vi "ChangePBTime.vi"(8 "Instruction to change":i32, 9 "Time":dbl, 10 "Input parameters":T2) -> (1 "Time out":dbl, 2 "output parameters":T2)   [LabVIEW 2013]
uses:
  6704/6704_static_voltages_control.ctl
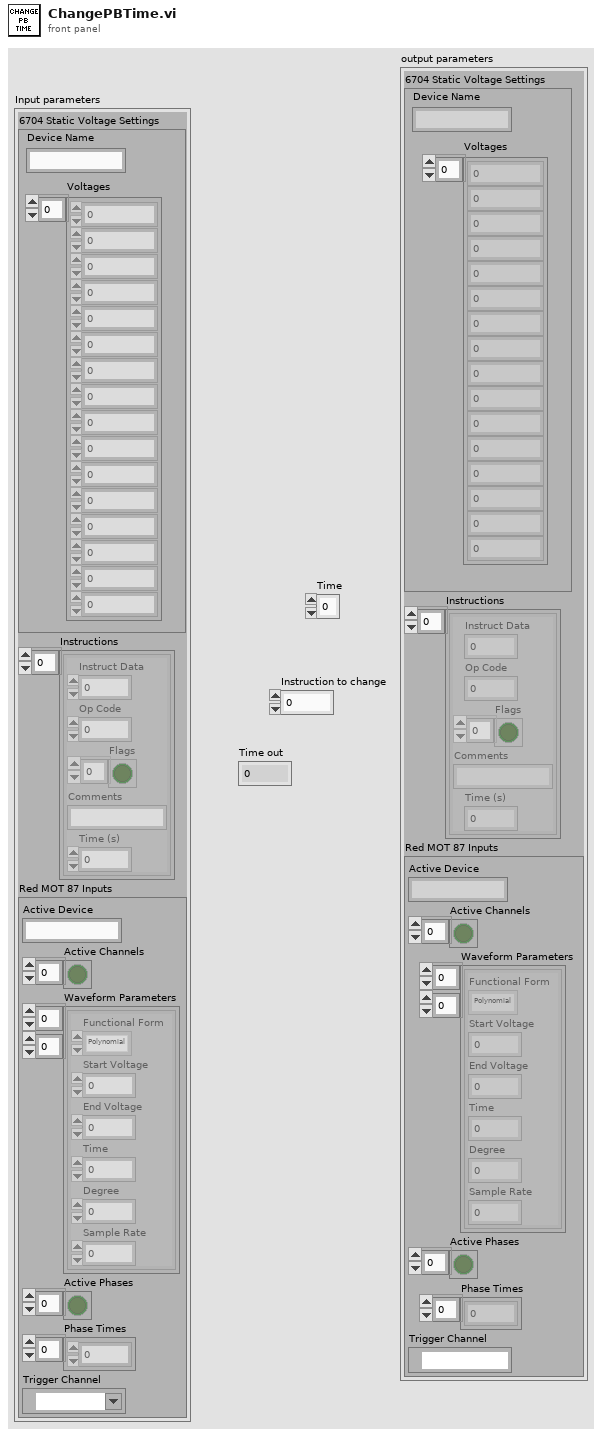
[diagram p1: front panel]
types:
  T1 = typedef "6704_static_voltages_control.ctl" = cluster{"Device Name":string, "Voltages":dbl[]}
  T2 = cluster{"6704 Static Voltage Settings":T1, "Instructions":cluster{"Instruct Data":i32, "Op Code":i32, "Flags":bool[], "Comments":string, "Time (s)":dbl}[], "Red MOT 87 Inputs":cluster{"Active Device":string, "Active Channels":bool[], "Waveform Parameters":cluster{"Functional Form":enum16{"Polynomial", "Exponential"}, "Start Voltage":dbl, "End Voltage":dbl, "Time":dbl, "Degree":i8, "Sample Rate":dbl}[][], "Active Phases":bool[], "Phase Times":dbl[], "Trigger Channel":tag}}
  T3 = cluster{"Instruct Data":i32, "Op Code":i32, "Flags":bool[], "Comments":string, "Time (s)":dbl}[]
  T4 = cluster{"Instruct Data":i32, "Op Code":i32, "Flags":bool[], "Comments":string, "Time (s)":dbl}
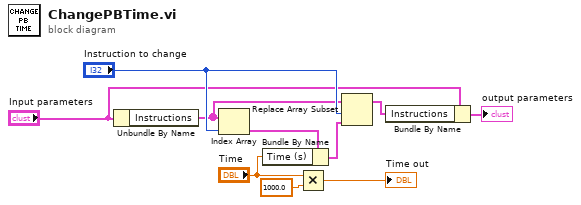
[diagram p0: block diagram]
diagram:
  n1 = Unbundle By Name("Input parameters") -> ("Instructions"=w4:T3)
  n2 = Index Array(array=w4, index="Instruction to change") -> (element=w8:T4)
  n3 = Bundle By Name(cluster=w8, "Time (s)"="Time") -> (w6:T4)
  n4 = Multiply(x="Time", y=1000.0) -> (x*y=→"Time out":dbl)
  n5 = Replace Array Subset(array=w4, new element=w6, index="Instruction to change") -> (w3:T3)
  n6 = Bundle By Name(cluster="Input parameters", "Instructions"=w3) -> (→"output parameters":T2)
